vi "Home all Axes.vi"(8 "error in (no error)":errorcluster) -> (0 "error out":errorcluster)   [LabVIEW 2019, in "ESP301.lvlib"]
uses:
  ESP301.lvlib
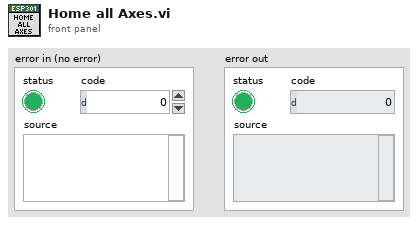
[diagram p1: front panel]
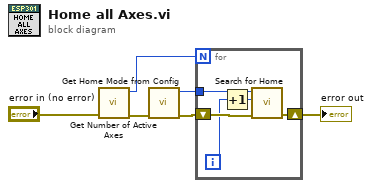
[diagram p0: block diagram]
diagram:
  n1 = call "Get Number of Active Axes.vi"("error in (no error)"="error in (no error)") -> ("error out"=w4:errorcluster, "value"=w6:i32)  [unwired: 9 in]
  n2 = call "Get Home Mode from Config.vi"("error in (no error)"=w4) -> ("error out"=w5:errorcluster, "Home Mode"=w2:i32)  [unwired: 9 in]
  n3 = for {
    N: w6 -> [_]
    tunnel: w2 -> [w10]
    shift-right: [w11] -> w1
    shift-left: w5 -> [w9]
    i -> [w8]
    n4 = Increment(x=w8) -> (x+1=w7:i32)
    n5 = call "Search for Home.vi"("error in (no error)"=w9, "Axis"=w7, "Home Mode"=w10) -> ("error out"=w11:errorcluster)  [unwired: 8 in]
  }
  "error out" <- w1
